vi "Create Publish Data Events.vi"(8 "error in (no error)":errorcluster, 11 "UserEvents in":refnum<class "User Events.lvclass">) -> (0 "error out":errorcluster, 3 "UserEvents out":refnum<class "User Events.lvclass">)   [LabVIEW 2016, in "User Events.lvclass"]
uses:
  User Events.lvclass
  Typedefs/StateTypes.ctl
  Typedefs/ScanProgress.ctl
  Typedefs/ActuatorData.ctl
  Typedefs/AllTestStatus.ctl
  Typedefs/TestStatus.ctl
  User Events.lvclass/User Events.ctl
  Typedefs/HPMT_Typedefs.lvlib
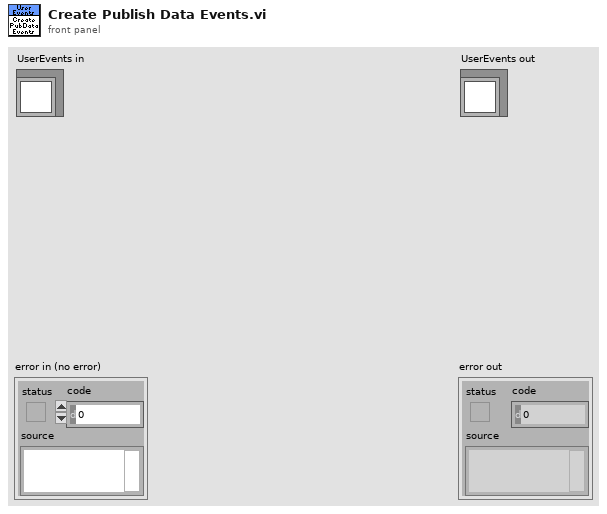
[diagram p1: front panel]
types:
  T1 = typedef "HPMT_Typedefs.lvlib/ActuatorData.ctl" = cluster{"Timestamp":dbl, "Force":dbl, "Encoder Value":i32, "Displacement Sensor 1":dbl, "Displacement Sensor 2":dbl}
  T2 = typedef "HPMT_Typedefs.lvlib/AllTestStatus.ctl" = cluster{"Stiffness Test":T3}
  T3 = typedef "HPMT_Typedefs.lvlib/TestStatus.ctl" = enum16{"Not Run", "Running", "Passed", "Failed"}
  T4 = typedef "HPMT_Typedefs.lvlib/ScanProgress.ctl" = cluster{"Actuator Data":T1}
  T5 = typedef "HPMT_Typedefs.lvlib/StateTypes.ctl" = enum16{"Offline State", "Fault State", "Standby State", "Disabled State", "Enabled State", "Wait For User Input State", "Test Actuator State"}
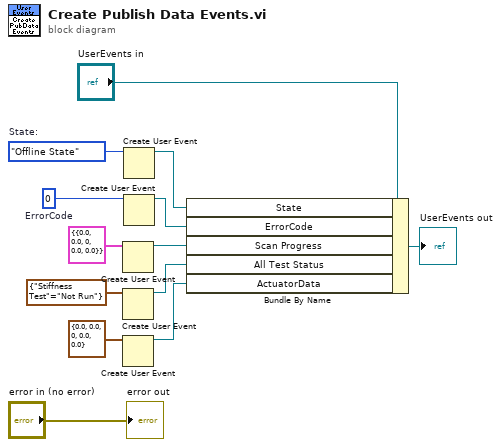
[diagram p0: block diagram]
diagram:
  w9 = 0  # ErrorCode
  w10 = StateTypes."Offline State"  # State:
  n1 = Create User Event(user event datatype=T4 {"Actuator Data"={"Timestamp"=0.0, "Force"=0.0, "Encoder Value"=0, "Displacement Sensor 1"=0.0, "Displacement Sensor 2"=0.0}} ("Chart Data")) -> (user event=w5:refnum<user-event>)  [unwired: 1 in, 1 out]
  n2 = Create User Event(user event datatype=T2 {"Stiffness Test"=enum."Not Run"} ("AllTestStatus")) -> (user event=w3:refnum<user-event>)  [unwired: 1 in, 1 out]
  n3 = Create User Event(user event datatype=T1 {"Timestamp"=0.0, "Force"=0.0, "Encoder Value"=0, "Displacement Sensor 1"=0.0, "Displacement Sensor 2"=0.0} ("Actuator Data")) -> (user event=w1:refnum<user-event>)  [unwired: 1 in, 1 out]
  n4 = Create User Event(user event datatype=w10) -> (user event=w8:refnum<user-event>)  [unwired: 1 in, 1 out]
  n5 = Create User Event(user event datatype=w9) -> (user event=w7:refnum<user-event>)  [unwired: 1 in, 1 out]
  n6 = Bundle By Name(cluster="UserEvents in", "State"=w8, "ErrorCode"=w7, "Scan Progress"=w5, "All Test Status"=w3, "ActuatorData"=w1) -> (→"UserEvents out":refnum<class "User Events.lvclass">)
  "error out" <- "error in (no error)"
